vi "Set CAN_Raw.vi"(8 "error in (no error)":errorcluster, 9 "Data":u8[](array[numeric]), 10 "Identifier":u32, 11 "Connection Info":T1) -> (0 "error out":errorcluster, 3 "Connection Info":T1)   [LabVIEW 2015, in "J1939 Host Automation API.lvlib"]
uses:
  J1939 Host Automation API.lvlib
  Shared/STM/TCP/stm_TCP Connection Info.ctl
  Shared/STM/_SubVIs/stm_MetaDataElement.ctl
  Shared/J1939 Utilities/Types/CAN Outgoing Message Cluster.ctl
  Shared/J1939 Addon Shared.lvlib
  Shared/J1939 Utilities/J1939 Utilities.lvlib
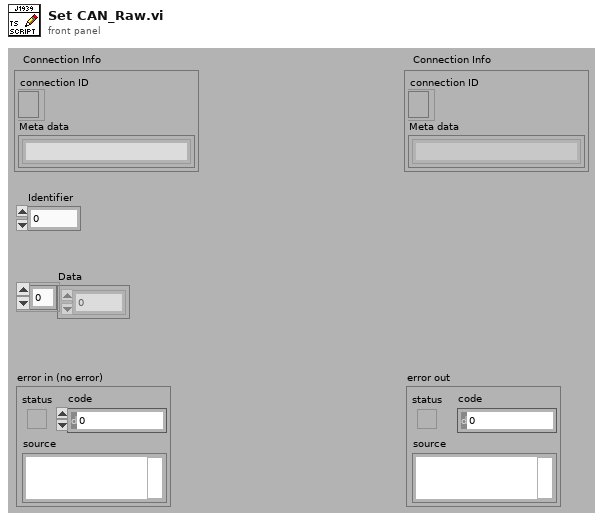
[diagram p1: front panel]
types:
  T1 = typedef "J1939 Addon Shared.lvlib/stm_TCP Connection Info.ctl" = cluster{"connection ID":refnum<k5>, "Meta data":T2[]}
  T2 = typedef "J1939 Addon Shared.lvlib/stm_MetaDataElement.ctl" = string
  T3 = typedef "J1939 Addon Shared.lvlib/J1939 Utilities.lvlib/CAN Outgoing Message Cluster.ctl" = cluster{"Identifier":u32, "Data":u8[]}
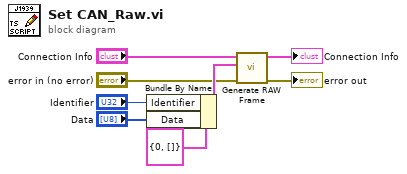
[diagram p0: block diagram]
diagram:
  n1 = Bundle By Name(cluster=T3 {"Identifier"=0, "Data"=[]} ("Data to Send"), "Identifier"="Identifier", "Data"="Data") -> (w5:T3)
  n2 = call "Generate RAW Frame.vi"("error in (no error)"="error in (no error)", "Data to Send"=w5, "Connection Info"="Connection Info") -> ("error out"=→"error out":errorcluster, "Connection Info Out"=→"Connection Info":T1)  [unwired: 7 in]
